vi "OAT Tachless Refine Speed Profile.vi"(4 "TF Plot Ref":refnum<vi>, 5 "Chkpnt Order":dbl format="%.2f", 6 "Time Boundary":cluster{"Time 1":dbl, "Time 2":dbl} {"Time 2" format="%.2f"; "Time 1" format="%.2f"}, 7 "sampling frequency [Hz]":dbl=1.0 format="%.2f", 8 "bandwidth":T3={"bandwidth value"=0.5, "bandwidth unit"=enum."Order"} {"bandwidth value" min=0.0 format="%.2f"}, 9 "interested orders list":dbl[](array[numeric]) format="%.2f", 10 "refined profile":T2 {"speed [RPM]" format="%.2f"; "time [s]" format="%.2f"}, 11 "RefNum":T1) -> (2 "refined profile":T2 {"speed [RPM]" format="%.2f"; "time [s]" format="%.2f"})   [LabVIEW 2017, in "SoundVib_Tachless.lvlib"]
uses:
  <vilib>/addons/Sound and Vibration/Order Analysis/Tachless/SoundVib_Tachless.lvlib
  <vilib>/addons/Sound and Vibration/Order Analysis/Tach Process/SubVIs/speed profile.ctl
  <vilib>/addons/Sound and Vibration/Order Analysis/Ref Gabor Order Tracking/Mask Bandwidth.ctl
  <vilib>/addons/Sound and Vibration/Order Analysis/Ref Gabor Order Tracking/GT RefNum.ctl
  <vilib>/addons/Sound and Vibration/Order Analysis/Ref Gabor Order Tracking/window information.ctl
  <vilib>/addons/Sound and Vibration/Order Analysis/Ref Gabor Order Tracking/Get Freq-Time Spectral Map (DBL).vi
  <vilib>/addons/Sound and Vibration/Order Analysis/Gabor Order Tracking/SoundVib_Gabor.lvlib
  <vilib>/Analysis/NI_AALBase.lvlib
  <vilib>/addons/Sound and Vibration/Order Analysis/Tach Process/SoundVib_TachProcess.lvlib
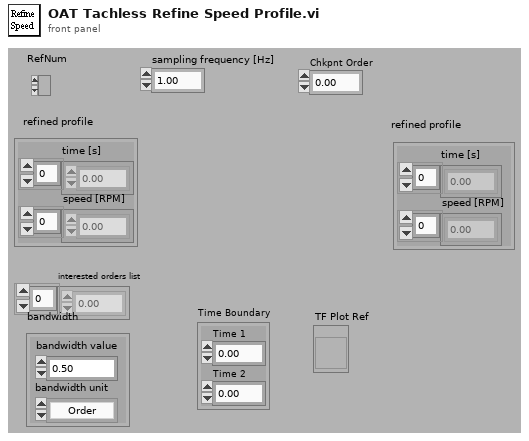
[diagram p1: front panel]
types:
  T1 = typedef "SoundVib_Gabor.lvlib/GT RefNum.ctl" = refnum<k1>
  T2 = typedef "SoundVib_TachProcess.lvlib/speed profile.ctl" = cluster{"time [s]":dbl[], "speed [RPM]":dbl[]}
  T3 = typedef "SoundVib_Gabor.lvlib/Mask Bandwidth.ctl" = cluster{"bandwidth value":dbl, "bandwidth unit":enum16{"Order", "Hz"}}
  T4 = typedef "SoundVib_Gabor.lvlib/window information.ctl" = cluster{"window type":u32, "window length":i32}
  T5 = typedef "LVOffsetAndMultiplierTypeDef.ctl" = cluster{"Offset":dbl, "Multiplier":dbl}
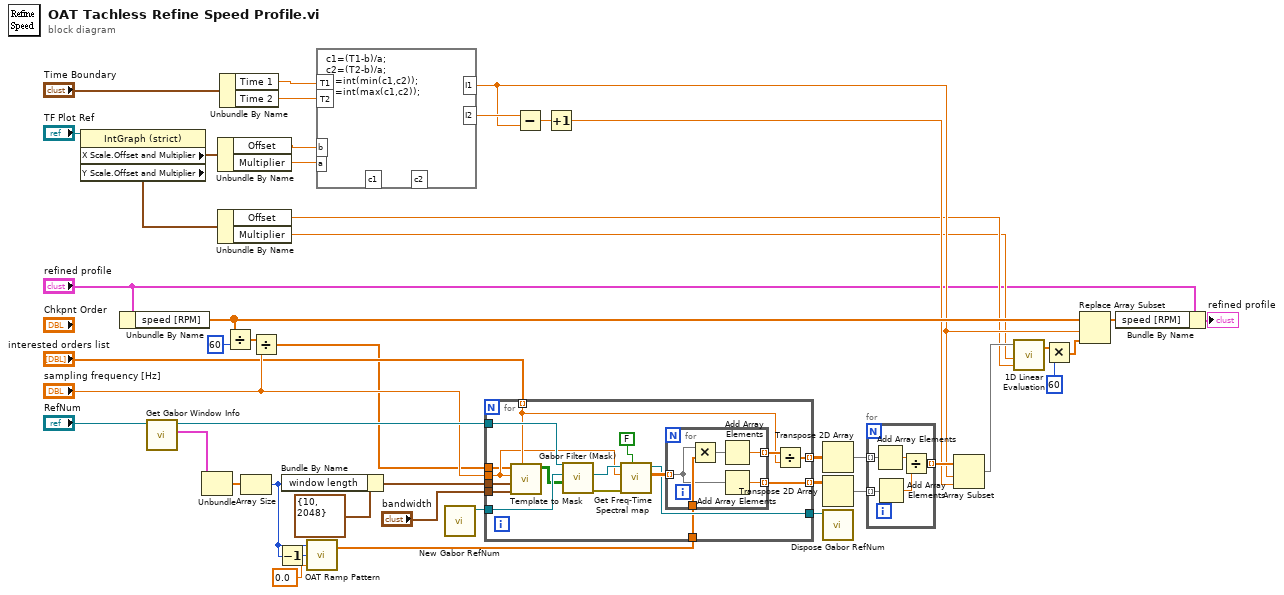
[diagram p0: block diagram]
diagram:
  n1 = property on="Property Node" class="IntGraph (strict)"(reference="TF Plot Ref") -> ("X Scale.Offset and Multiplier"=w38:T5, "Y Scale.Offset and Multiplier"=w37:T5)  [unwired: 1 in, 2 out]
  n2 = Unbundle By Name("refined profile") -> ("speed [RPM]"=w23:dbl[])
  n3 = call <vilib>:"Get Gabor Window Info.vi"("RefNum in"="RefNum") -> ("analysis window"=w35:cluster{"gamma[i]":dbl[], "dM":i32, "N":i32}, "RefNum out"=w30:T1)  [unwired: 7 in, 2 out]
  n4 = Unbundle(w35) -> ("gamma[i]"=w34:dbl[])  [unwired: 2 out]
  n5 = Unbundle By Name(w38) -> ("Offset"=w43:dbl, "Multiplier"=w44:dbl)
  n6 = Unbundle By Name(w37) -> ("Offset"=w18:dbl, "Multiplier"=w8:dbl)
  n7 = Unbundle By Name("Time Boundary") -> ("Time 1"=w41:dbl, "Time 2"=w40:dbl)
  n8 = Divide(x=w23, y=60) -> (x/y=w7:dbl[])
  n9 = Array Size(array=w34) -> (size(s)=w11:i32)
  n10 = Divide(x=w7, y="sampling frequency [Hz]") -> (x/y=w2:dbl[])
  n11 = Decrement(x=w11) -> (x-1=w12:i32)
  n12 = Bundle By Name(cluster=T4 {"window type"=10, "window length"=2048} ("window info"), "window length"=w11) -> (w32:T4)
  n13 = call <vilib>:"OAT Ramp Pattern.vi"("start"=0.0, "end"=w12, "samples"=w11) -> ("Ramp Pattern"=w9:dbl[])  [unwired: 1 out]
  n14 = formula code="c1=(T1-b)/a;\nc2=(T2-b)/a;\nI1=int(min(c1,c2));\nI2=int(max(c1,c2));"("T1"=w41, "T2"=w40, "a"=w44, "b"=w43) -> ("I1"=w20:dbl, "I2"=w25:dbl)  [unwired: 2 out]
  n15 = call <vilib>:"New Gabor RefNum.vi"() -> ("RefNum"=w29:T1)  [unwired: 9 in, 1 out]
  n16 = for {
    tunnel: "interested orders list" -> [w53] mode=indexing
    tunnel: "sampling frequency [Hz]" -> [w49]
    tunnel: w32 -> [w62]
    tunnel: "bandwidth" -> [w61]
    tunnel: w30 -> [w57]
    tunnel: w29 -> [w56]
    tunnel: [w52] -> w28 mode=indexing
    tunnel: [w51] -> w26
    tunnel: w9 -> [w50]
    tunnel: [w47] -> w5 mode=indexing
    tunnel: w2 -> [w46]
    n17 = call <vilib>:"Template to Mask.vi"("order (1.0)"=w53, "bandwidth"=w61, "window info"=w62, "sampling frequency [S/s]"=w49, "Gabor template"=w46) -> ("mask array"=w48:bool[][])  [unwired: 6 in]
    n18 = call <vilib>:"Gabor Filter (Mask).vi"("mask array"=w48, "dest RefNum in"=w56, "src RefNum in"=w57) -> ("error out"=w60:errorcluster, "dest RefNum out"=w58:T1)  [unwired: 6 in, 1 out]
    n19 = call-poly <vilib>:"Get Freq-Time Spectral map.vi"("dB On (T)"=FALSE, "error in (no error)"=w60, "sampling frequency [Hz]"=w49, "RefNum in"=w58) -> ("spectral map"=w55:dbl[][], "RefNum out"=w51:T1)  [unwired: 2 in, 4 out]
    n20 = for {
      tunnel: w55 -> [w65] mode=indexing
      tunnel: [w64] -> w54 mode=indexing
      tunnel: w50 -> [w67]
      tunnel: [w63] -> w47 mode=indexing
      n21 = Multiply(x=w65, y=w67) -> (x*y=w66:dbl[])
      n22 = Add Array Elements(numeric array=w66) -> (sum=w64:dbl)
      n23 = Add Array Elements(numeric array=w65) -> (sum=w63:dbl)
    }
    n24 = Divide(x=w54, y=w53) -> (x/y=w52:dbl[])
  }
  n25 = Subtract(x=w25, y=w20) -> (x-y=w24:dbl)
  n26 = Increment(x=w24) -> (x+1=w21:dbl)
  n27 = Transpose 2D Array(2D array=w28) -> (transposed array=w27:dbl[][])
  n28 = Transpose 2D Array(2D array=w5) -> (transposed array=w4:dbl[][])
  n29 = call <vilib>:"Dispose Gabor RefNum.vi"("RefNum in"=w26) -> ()  [unwired: 7 in, 1 out]
  n30 = for {
    tunnel: w27 -> [w70] mode=indexing
    tunnel: [w71] -> w22 mode=indexing
    tunnel: w4 -> [w72] mode=indexing
    n31 = Add Array Elements(numeric array=w70) -> (sum=w68:dbl)
    n32 = Add Array Elements(numeric array=w72) -> (sum=w69:dbl)
    n33 = Divide(x=w68, y=w69) -> (x/y=w71:dbl)
  }
  n34 = Array Subset(array=w22, index=w20, length=w21) -> (w19:dbl[])
  n35 = call <vilib>:"1D Linear Evaluation.vi"("offset"=w18, "scale"=w8, "X"=w19) -> ("Y[i]=X[i]*a+b"=w17:dbl[])  [unwired: 1 out]
  n36 = Multiply(x=w17, y=60) -> (x*y=w15:dbl[])
  n37 = Replace Array Subset(array=w23, new element=w15, index=w20) -> (w14:dbl[])
  n38 = Bundle By Name(cluster="refined profile", "speed [RPM]"=w14) -> (→"refined profile":T2)
